vi "read_ini_file_string.vi"(8 "error in (no error)":errorcluster, 9 "key":string="UUTFWChecksum_Pri", 10 "section":string="MAS80W", 11 "configuration file path":path=path "C:/Project/SolaHD_FCT/Configuration/config.ini") -> (0 "error out":errorcluster, 1 "found?":bool, 2 "value":string)   [LabVIEW 2016]
uses:
  <vilib>/Utility/config.llb/Read Key (String).vi
  <vilib>/Utility/config.llb/NI_LVConfig.lvlib
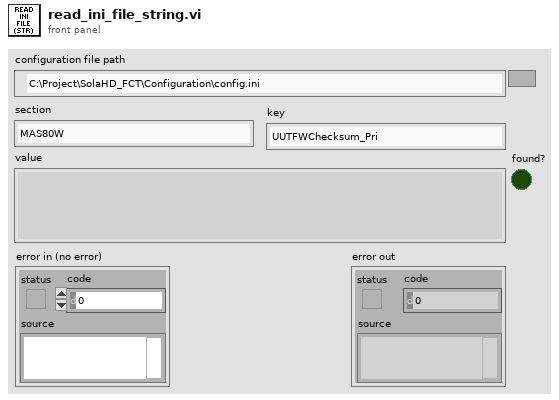
[diagram p1: front panel]
types:
  T1 = typedef "NI_LVConfig.lvlib/Config Data RefNum.ctl" = refnum<k1>
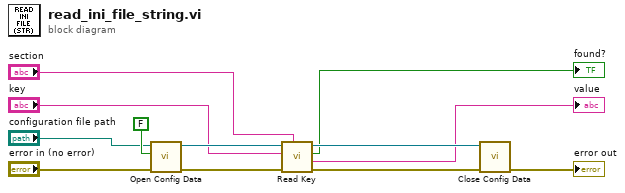
[diagram p0: block diagram]
diagram:
  n1 = call <vilib>:"Open Config Data.vi"("error in (no error)"="error in (no error)", "create file if necessary (T)"=FALSE, "configuration file path"="configuration file path") -> ("error out"=w7:errorcluster, "refnum"=w5:T1)  [unwired: 6 in, 1 out]
  n2 = call-poly <vilib>:"Read Key.vi"("section"="section", "error in (no error)"=w7, "key"="key", "refnum"=w5) -> ("error out"=w6:errorcluster, "value"=→"value":string, "found?"=→"found?":bool, "refnum out"=w8:T1)  [unwired: 4 in]
  n3 = call <vilib>:"Close Config Data.vi"("error in (no error)"=w6, "refnum"=w8) -> ("error out"=→"error out":errorcluster)  [unwired: 8 in, 1 out]
